vi "ZMC Open Pci.vi"(8 "error in (no error)":errorcluster caption="错误输入（无错误）", 10 "phandle":u32, 11 "cardnum":u32) -> (0 "error out":errorcluster caption="错误输出", 2 "phandle out":u32, 3 "function return":i32)   [LabVIEW 2015, in "zauxdll.lvlib"]
doc: "int32 __stdcall ZMC_OpenPci(uint32 cardnum, ZMC_HANDLE * phandle);"
uses:
  zauxdll.lvlib
  zmotion.dll
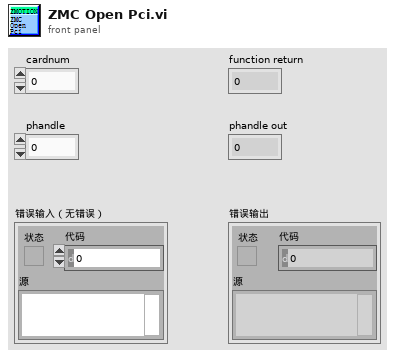
[diagram p1: front panel]
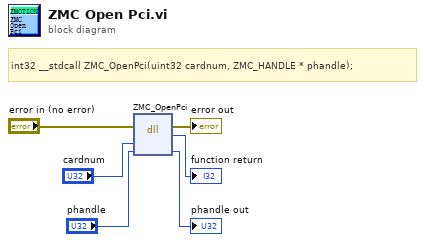
[diagram p0: block diagram]
diagram:
  # "int32 __stdcall ZMC_OpenPci(uint32 cardnum, ZMC_HANDLE * phandle);"
  n1 = dll-call lib="C:/Users/VIC/Desktop/GOGORO_SA/system/LLB/zmotion/zaux/zmotion.*" fn="ZMC_OpenPci"(error in="error in (no error)", "cardnum"="cardnum", "phandle"="phandle") -> (error out=→"error out":errorcluster, →"function return":i32, "phandle"=→"phandle out":u32)  [unwired: 3 in, 1 out]
